vi "TempMaster.vi"() -> (1 "TempQ":refnum<queue>, 2 "ScanQ":refnum<queue>, 3 "SweepQ":refnum<queue>)   [LabVIEW 2025]
uses:
  CTL's/Scan_Params (QMH).ctl
  Temp Cntrl.ctl
  TEMP_SWEEPER.ctl
panel:
  out "error out":errorcluster
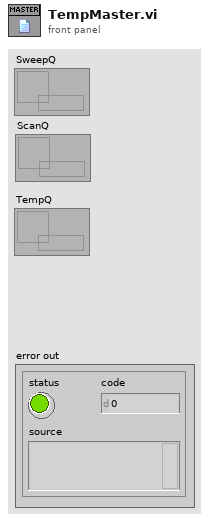
[diagram p1: front panel]
types:
  T1 = typedef "TEMP_SWEEPER.ctl" = cluster{"Temps(K)":dbl[], "Sweep States":enum16{"SET TEMP", "SWEEP IDLE", "NEXT TEMP", "SWEEP DONE"}}
  T2 = typedef "Temp Cntrl.ctl" = cluster{"Range (0:Off)":u16, "Manual Output (0.00 %)":dbl, "Rate (D) (0.0 %)":dbl, "Reset (I) (20.0)":dbl, "Gain (P) (50.0)":dbl, "Power Up Enable (F: Disable)":bool, "Max User Current (2.000)":dbl, "Heater Resistance (1:25 Ohms)":u16, "Max Current (0:User Specified)":u16, "Heater Out Display (1:Current)":u16, "Mode (0:Off)":u16, "Input (0:None)":u16, "Target Temp (K)":dbl, "Serial Configuration":cluster{"Baud Rate":u32, "Parity":u16, "Data Bits":u16, "Stop Bits":u16, "Flow Control":u16}, "VISA resource name":refnum<visa-resource-name>, "Configure Control Parameters (0: Configure)":u16, "Enable Setpoint (F:Disable)":bool, "Input (0:A)":u16, "Data Source (0:Kelvin)":u16, "Output's Control Loop (1:1)":u16, "STND DEV Threshold ":dbl, "Mean Tolerance ":dbl, "Current State":enum16{"1. INIT TEMP", "2. TC ON", "3. POLL_TEMPS", "4. TEMP_STAB", "5. TC IDLE", "6. APPLY NEXT TEMP", "7. TC OFF (Reset)"}}
  T3 = typedef "Scan_Params (QMH).ctl" = cluster{"Setpoint (I)":dbl[], "Bias (V)":dbl[], "Number of scans":u8, "Port number (3364)":u32, "Avoid zero threshold (V)":dbl, "Current State":enum16{"1. BIAS", "2. INIT_SCAN", "3. SCAN_IDLE", "4. INTER_SCAN", "5. NEW_COORDS_&_FRAME", "6. FINAL_SCAN", "7. POLL_BIAS", "8. Z-CONT", "9. STOP"}}
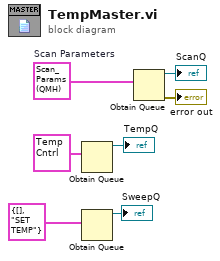
[diagram p0: block diagram]
diagram:
  w7 = T3 {"Setpoint (I)"=[], "Bias (V)"=[], "Number of scans"=1, "Port number (3364)"=3364, "Avoid zero threshold (V)"=0.004999999888241291, "Current State"=enum."2. INIT_SCAN"}  # Scan Parameters
  n1 = Obtain Queue(element data type=T2 {"Range (0:Off)"=0, "Manual Output (0.00 %)"=0.0, "Rate (D) (0.0 %)"=0.0, "Reset (I) (20.0)"=20.0, "Gain (P) (50.0)"=50.0, "Power Up Enable (F: Disable)"=FALSE, "Max User Current (2.000)"=2.0, "Heater Resistance (1:25 Ohms)"=1, "Max Current (0:User Specified)"=0, "Heater Out Display (1:Current)"=1, "Mode (0:Off)"=0, "Input (0:None)"=0, "Target Temp (K)"=0.0, "Serial Configuration"={"Baud Rate"=57600, "Parity"=1, "Data Bits"=7, "Stop Bits"=10, "Flow Control"=0}, "VISA resource name"="", "Configure Control Parameters (0: Configure)"=0, "Enable Setpoint (F:Disable)"=FALSE, "Input (0:A)"=0, "Data Source (0:Kelvin)"=0, "Output's Control Loop (1:1)"=1, "STND DEV Threshold "=0.1, "Mean Tolerance "=0.02, "Current State"=enum."1. INIT TEMP"} ("Temp Controller")) -> (queue out=→"TempQ":refnum<queue>)  [unwired: 4 in, 2 out]
  n2 = Obtain Queue(element data type=T1 {"Temps(K)"=[], "Sweep States"=enum."SET TEMP"} ("Temp and Field Range")) -> (queue out=→"SweepQ":refnum<queue>)  [unwired: 4 in, 2 out]
  n3 = Obtain Queue(element data type=w7) -> (queue out=→"ScanQ":refnum<queue>, error out=→"error out":errorcluster)  [unwired: 4 in, 1 out]
